vi "LAC Cmd130R_LD Auto_adj result.vi"(7 "timeout(ms)":u32, 8 "error in":errorcluster, 11 "VISA name in":refnum<visa-resource-name>) -> (0 "error out":errorcluster, 1 "readout":string, 3 "VISA name out":refnum<visa-resource-name>)   [LabVIEW 8.6]
panel:
  # "readout items\n\n¨0〃=OFF or Not adjusted, \n¨1〃=Under automatic adjustment, \n¨2〃=Successful automatic adjustment, \n¨3〃=Failed automatic adjustment"
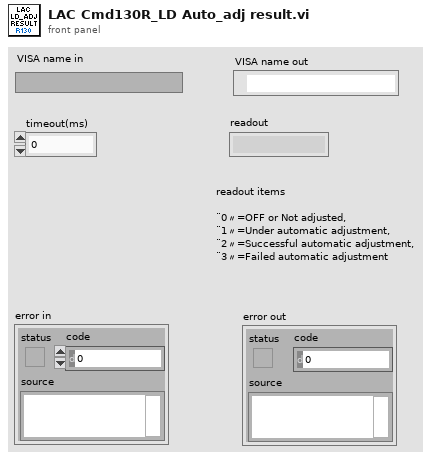
[diagram p1: front panel]
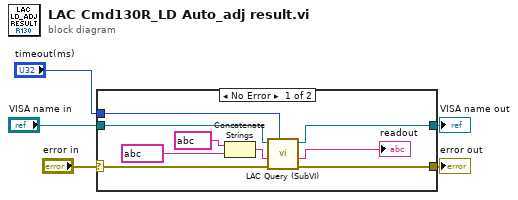
[diagram p0: block diagram]
diagram:
  n1 = case shown="No Error" "error in" {
    selector: "error in" -> [w10 w16]
    tunnel: "VISA name in" -> [w12 w15]
    tunnel: [w14 w15] -> w4
    tunnel: [w13 w16] -> w3
    tunnel: "timeout(ms)" -> [w11 _]
    frame #0 {
      n2 = Concatenate Strings(string ? ("string"), string ? ("write buffer")) -> (w8:string)
      n3 = call "LAC Query (SubVI).vi"("timeout(ms)"=w11, "error in"=w10, "Command"=w8, "VISA name in"=w12) -> ("error out"=w13:errorcluster, "read buffer"=→"readout":string, "VISA name out"=w14:refnum<visa-resource-name>)  [unwired: 5 in]
    }
    frame #1 {
    }
  }
  "VISA name out" <- w4
  "error out" <- w3
